vi "Tag Channel Example - Almost Right.vi"() -> ()   [LabVIEW 2023]
doc: "This VI demonstrates how to use the Tag to represent a configuration value that is set initially but may be changed by the user while the program is running. That new configuration value is immediately communicated to several running processes that need to know about the changed value.\n\nThe VI looks like it works, but there are some very subtle problems lurking in this code."
uses:
  <extravilib>/ChannelInstances/Tag-u32/Instantiate.vi
  <extravilib>/ChannelInstances/Tag-u32/Endpoint.vi
  <extravilib>/ChannelInstances/Tag-u32/EndpointRead.vi
  <extravilib>/ChannelInstances/Tag-u32.lvlib
panel:
  out "C above threshold?":bool
  out "Thermometer C":dbl(slide) scale=0.0..10.0
  out "B above threshold?":bool
  out "Thermometer B":dbl(slide) scale=0.0..10.0
  out "A above threshold?":bool
  out "Thermometer A":dbl(slide) scale=0.0..10.0
  in  "Threshold Setting":u32(slide)=5 scale=0.0..10.0
  in  "Stop":bool
  # "Overview: Demonstrates how to use the Tag, which is one of the channel wire templates that ships with LabVIEW.  Tags work like variables (local, global, or shared) insofar as they represent a single value that can be written to or read from many points in the application. The advantage of a Tag is that all of the writers and readers can be found by tracing the wire into its various subVIs, so you never have to worry about some unknown part of your application accessing the value erroneously.\nYou should already be aware of the basics of channels generally to fully understand this example.\n\nInstructions:\n1. Run the VI. \n2. While running, change the Threshold Setting. Notice the thermometers immediately start using the new setting for their \"Too hot!\" indicators.\n3. Press the Stop button.\n4. Review the comments on the block diagram."
  # "When this VI is running, any time a thermometer is warmer than the Threshold Setting, that thermometer should say \"Too hot!\" in the Boolean at the bottom."
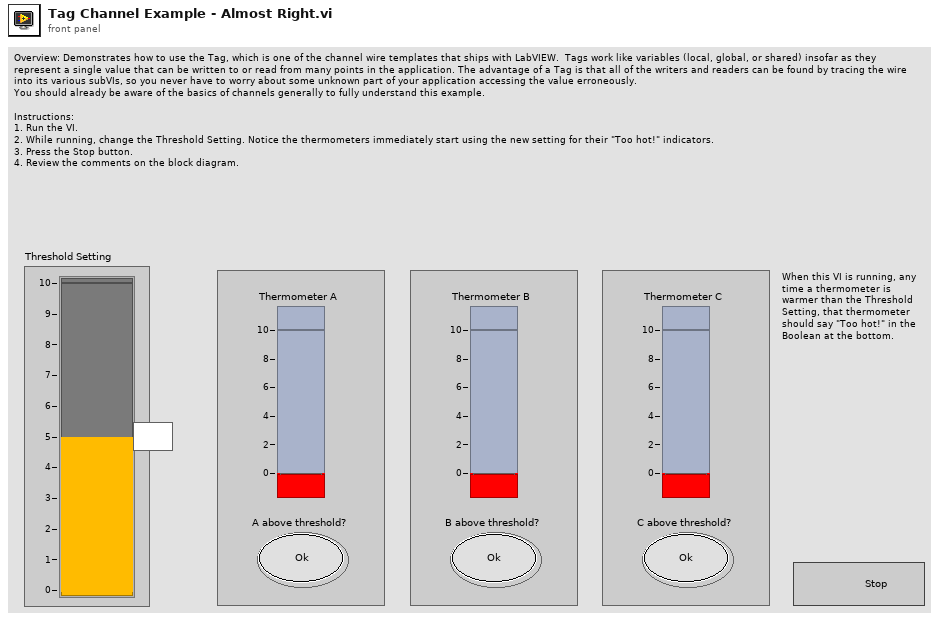
[diagram p1: front panel]
types:
  T1 = typedef "Tag-u32.lvlib/))Channel.ctl" = refnum<queue>
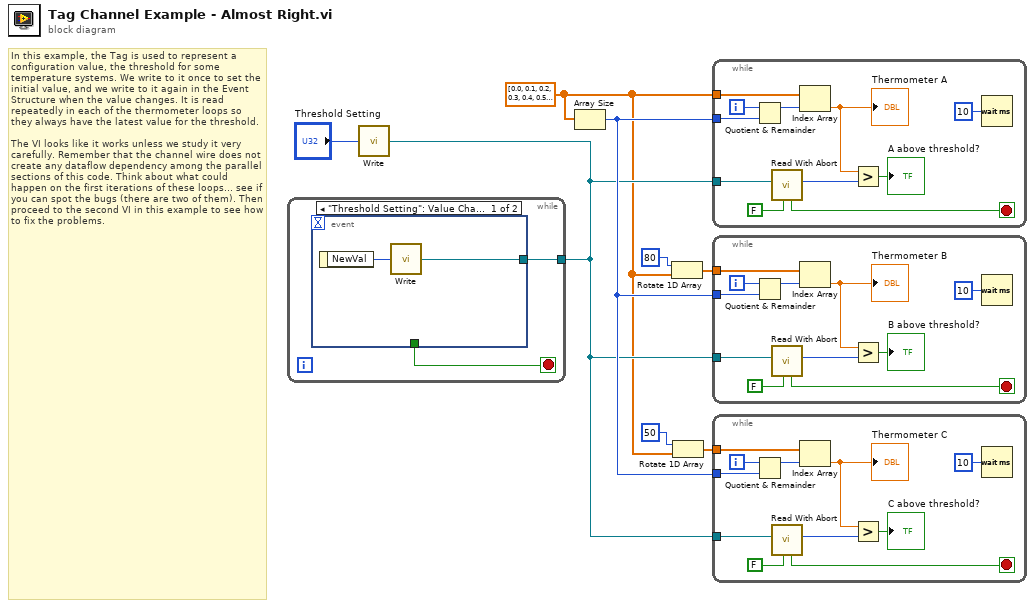
[diagram p0: block diagram]
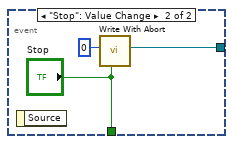
[diagram p2: hidden frame]
diagram:
  w3 = dbl[] [0.0, 0.1, 0.2, 0.3, 0.4, 0.5, 0.6, 0.7, 0.8, 0.9, 1.0, 1.1, 1.2, 1.3, 1.4, 1.5, 1.6, 1.7, 1.8, 1.9, 2.0, 2.1, 2.2, 2.3, 2.4, 2.5, 2.6, 2.7, 2.8, 2.9, 3.0, 3.1, 3.2, 3.3, 3.4, 3.5, 3.6, 3.7, 3.8, 3.9, 4.0, 4.1, 4.2, 4.3, 4.4, 4.5, 4.6, 4.7, 4.8, 4.9, 5.0, 5.1, 5.2, 5.3, 5.4, 5.5, 5.6, 5.7, 5.8, 5.9, 6.0, 6.1, 6.2, 6.3, 6.4, 6.5, 6.6, 6.7, 6.8, 6.9, 7.0, 7.1, 7.2, 7.3, 7.4, 7.5, 7.6, 7.7, 7.8, 7.9, 8.0, 8.1, 8.2, 8.3, 8.4, 8.5, 8.6, 8.7, 8.8, 8.9, 9.0, 9.1, 9.2, 9.3, 9.4, 9.5, 9.6, 9.7, 9.8, 9.9, 10.0, 10.0, 9.9, 9.8, 9.7, 9.6, 9.5, 9.4, 9.3, 9.2, 9.1, 9.0, 8.9, 8.8, 8.7, 8.6, 8.5, 8.4, 8.3, 8.2, 8.1, 8.0, 7.9, 7.8, 7.7, 7.6, 7.5, 7.4, 7.3, 7.2, 7.1, 7.0, 6.9, 6.8, 6.7, 6.6, 6.5, 6.4, 6.3, 6.2, 6.1, 6.0, 5.9, 5.8, 5.7, 5.6, 5.5, 5.4, 5.3, 5.2, 5.1, 5.0, 4.9, 4.8, 4.7, 4.6, 4.5, 4.4, 4.3, 4.2, 4.1, 4.0, 3.9, 3.8, 3.7, 3.6, 3.5, 3.4, 3.3, 3.2, 3.1, 3.0, 2.9, 2.8, 2.7, 2.6, 2.5, 2.4, 2.3, 2.2, 2.1, 2.0, 1.9, 1.8, 1.7, 1.6, 1.5, 1.4, 1.3, 1.2, 1.1, 1.0, 0.9, 0.8, 0.7, 0.6, 0.5, 0.4, 0.3, 0.2, 0.1, 0.0] ("x/y")
  # "In this example, the Tag is used to represent a configuration value, the threshold for some temperature systems. We write to it once to set the initial value, and we write to it again in the Event Structure when the value changes. It is read repeatedly in each of the thermometer loops so they always have the latest value for the threshold.\n\nThe VI looks like it works unless we study it very carefully. Remember that the channel wire does not create any dataflow dependency among the parallel sections of this code. Think about what could happen on the first iterations of these loops... see if you can spot the bugs (there are two of them). Then proceed to the second VI in this example to see how to fix the problems."
  n1 = call <extravilib>:"Write.vi"("element"="Threshold Setting") -> ("channel"=w6:T1)  [unwired: 1 out]
  n2 = while {
    tunnel: w6 -> [w10]
    stop <- w9 stop-if-true
    n3 = event shown="[0] \"Threshold Setting\": Value Change" {
      selector: _ -> [_ _]
      dyn-events: _ -> [_ _]
      timeout: _ -> [_ _]
      tunnel: [w12 w15] -> w10
      tunnel: [_ "Stop"] -> w9
      event "Threshold Setting": Value Change {
        n4 = event-data() -> ("NewVal"=w11:u32)  [unwired: 1 in]
        n5 = call <extravilib>:"Write.vi"("element"=w11) -> ("channel"=w12:T1)  [unwired: 1 out]
      }
      event "Stop": Value Change {
        n6 = event-data() -> ()  [unwired: 1 in, 1 out]
        n7 = call <extravilib>:"Write With Abort.vi"("abort"="Stop", "element"=u32 0) -> ("channel"=w15:T1)  [unwired: 7 in, 2 out]
      }
    }
  }
  n8 = Array Size(array=w3) -> (size(s)=w7:i32)
  n9 = Rotate 1D Array(1:w3, 2:80 ("n")) -> (0:w2:dbl[])
  n10 = Rotate 1D Array(1:w3, 2:50 ("n")) -> (0:w5:dbl[])
  n11 = while {
    tunnel: w6 -> [w26]
    tunnel: w7 -> [w20]
    tunnel: w3 -> [w19]
    i -> [w21]
    stop <- w25 stop-if-true
    n12 = Quotient & Remainder(x=w21, y=w20) -> (x-y*floor(x/y)=w18:i32)  [unwired: 1 out]
    n13 = call <extravilib>:"Read With Abort.vi"("abort"=FALSE, "channel"=w26) -> ("element"=w24:u32, "aborted?"=w25:bool)  [unwired: 7 in, 1 out]
    n14 = Index Array(array=w19, index=w18) -> (element=w17:dbl)
    "Thermometer A" <- w17
    n15 = Greater?(x=w17, y=w24) -> (0:→"A above threshold?":bool)
    n16 = Wait (ms)(milliseconds to wait=u32 10) -> ()  [unwired: 1 out]
  }
  n17 = while {
    tunnel: w6 -> [w37]
    tunnel: w7 -> [w32]
    tunnel: w2 -> [w31]
    i -> [w33]
    stop <- w36 stop-if-true
    n18 = Quotient & Remainder(x=w33, y=w32) -> (x-y*floor(x/y)=w30:i32)  [unwired: 1 out]
    n19 = call <extravilib>:"Read With Abort.vi"("abort"=FALSE, "channel"=w37) -> ("element"=w35:u32, "aborted?"=w36:bool)  [unwired: 7 in, 1 out]
    n20 = Index Array(array=w31, index=w30) -> (element=w28:dbl)
    "Thermometer B" <- w28
    n21 = Greater?(x=w28, y=w35) -> (0:→"B above threshold?":bool)
    n22 = Wait (ms)(milliseconds to wait=u32 10) -> ()  [unwired: 1 out]
  }
  n23 = while {
    tunnel: w6 -> [w48]
    tunnel: w7 -> [w43]
    tunnel: w5 -> [w42]
    i -> [w44]
    stop <- w47 stop-if-true
    n24 = Quotient & Remainder(x=w44, y=w43) -> (x-y*floor(x/y)=w41:i32)  [unwired: 1 out]
    n25 = call <extravilib>:"Read With Abort.vi"("abort"=FALSE, "channel"=w48) -> ("element"=w46:u32, "aborted?"=w47:bool)  [unwired: 7 in, 1 out]
    n26 = Index Array(array=w42, index=w41) -> (element=w39:dbl)
    "Thermometer C" <- w39
    n27 = Greater?(x=w39, y=w46) -> (0:→"C above threshold?":bool)
    n28 = Wait (ms)(milliseconds to wait=u32 10) -> ()  [unwired: 1 out]
  }
